vi "FTW-Message-Request-Interpret.vi"(8 "error in":errorcluster, 11 "FTW Incoming Request":refnum<class "FTW-Message-IncomingRequest.lvclass">) -> (0 "error out":errorcluster, 1 "Request Body":string, 2 "Request Header":string, 3 "FTW Incoming Request out":refnum<class "FTW-Message-IncomingRequest.lvclass">)   [LabVIEW 2013, in "FTW-Actor.lvlib" / "FTW-Message-IncomingRequest.lvclass"]
uses:
  FTW-Message-IncomingRequest.lvclass
panel:
  # "Inputs"
  # "Outputs"
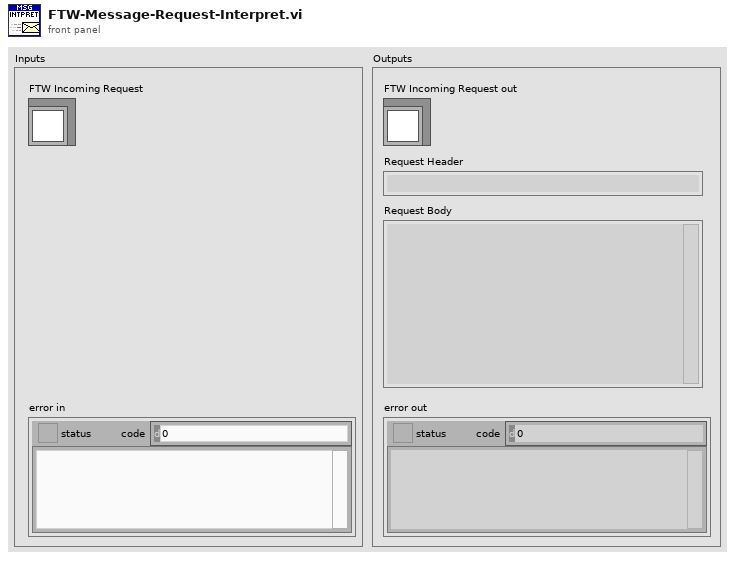
[diagram p1: front panel]
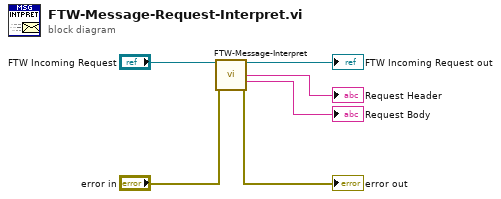
[diagram p0: block diagram]
diagram:
  n1 = call-dynamic "FTW-Message-Interpret.vi"("FTW Message"="FTW Incoming Request", "error in"="error in") -> ("FTW Message out"=→"FTW Incoming Request out":refnum<class "FTW-Message-IncomingRequest.lvclass">, "Message Header"=→"Request Header":string, "Message Body"=→"Request Body":string, "error out"=→"error out":errorcluster)  [unwired: 9 in, 1 out]
